vi "Flatten Value.vi"(8 "Error In":errorcluster, 11 "Int In":refnum<class "Int.lvclass">) -> (0 "Error Out":errorcluster, 1 "Value":string, 3 "Int Out":refnum<class "Int.lvclass">)   [LabVIEW 2020, in "NI_VIAnCFGDataStructure.lvlib" / "Int.lvclass"]
uses:
  <vilib>/addons/analyzer/VIAnCFGDataStructure/Data Types/Int/Int.lvclass
  <vilib>/addons/analyzer/VIAnCFGDataStructure/Data Types/Int/Int.lvclass/Int.ctl
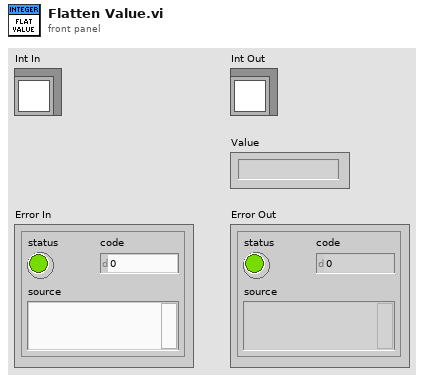
[diagram p1: front panel]
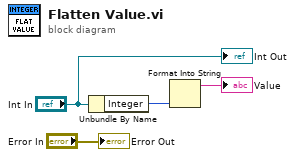
[diagram p0: block diagram]
diagram:
  n1 = Unbundle By Name("Int In") -> ("Integer"=w3:i64)
  n2 = Format Into String(w3) -> (resulting string=→"Value":string)  [unwired: 3 in, 1 out]
  "Int Out" <- "Int In"
  "Error Out" <- "Error In"
